vi "MGI Get Slope at Point.vi"(9 "Index":i32, 10 "Y[]":dbl[](array[numeric]), 11 "X[]":dbl[](array[numeric])) -> (3 "Slope Unit Vector[]":dbl[](array[numeric]))   [LabVIEW 2020]
doc: "Gets the unit length slope of the curve defined by the input arrays at the specified index.\n\nAuthored by Thomas E Henage\nsupport@mooregoodideas.com\nwww.mooregoodideas.com\n\nCopyright (c) 2010, Moore Good Ideas, Inc.\n\nAll rights reserved.\n\nRedistribution and use in source and binary forms, with or without modification, are permitted provided that the following conditions are met:\n\n * Redistributions of source code must retain the above copyright notice, this list of conditions and the following disclaimer.\n * Redistributions in binary form must reproduce the above copyright notice, this list of conditions and the following disclaimer in the documentation and/or other materials provided with the distribution.\n * Neither the name of Moore Good Ideas, Inc. nor the names of its contributors may be used to endorse or promote products derived from this software without specific prior written permission.\n\nTHIS SOFTWARE IS PROVIDED BY THE COPYRIGHT HOLDERS AND CONTRIBUTORS \"AS IS\" AND ANY EXPRESS OR IMPLIED WARRANTIES, INCLUDING, BUT NOT LIMITED TO, THE IMPLIED WARRANTIES OF MERCHANTABILITY AND FITNESS FOR A PARTICULAR PURPOSE ARE DISCLAIMED. IN NO EVENT SHALL THE COPYRIGHT OWNER OR CONTRIBUTORS BE LIABLE FOR ANY DIRECT, INDIRECT, INCIDENTAL, SPECIAL, EXEMPLARY, OR CONSEQUENTIAL DAMAGES (INCLUDING, BUT NOT LIMITED TO, PROCUREMENT OF SUBSTITUTE GOODS OR SERVICES; LOSS OF USE, DATA, OR PROFITS; OR BUSINESS INTERRUPTION) HOWEVER CAUSED AND ON ANY THEORY OF LIABILITY, WHETHER IN CONTRACT, STRICT LIABILITY, OR TORT (INCLUDING NEGLIGENCE OR OTHERWISE) ARISING IN ANY WAY OUT OF THE USE OF THIS SOFTWARE, EVEN IF ADVISED OF THE POSSIBILITY OF SUCH DAMAGE."
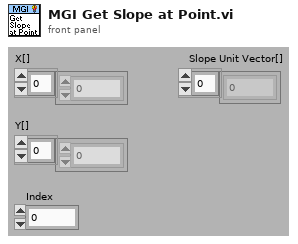
[diagram p1: front panel]
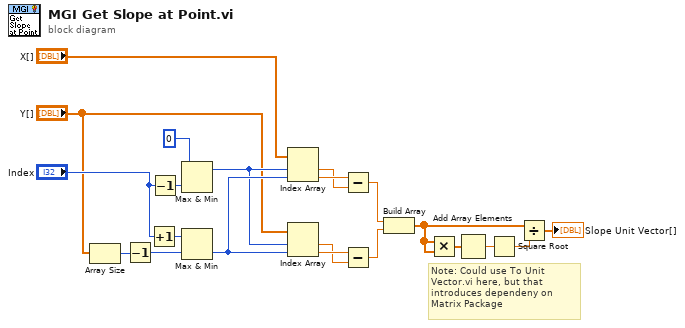
[diagram p0: block diagram]
diagram:
  # "Note: Could use To Unit Vector.vi here, but that introduces dependeny on Matrix Package"
  n1 = Array Size(array="Y[]") -> (size(s)=w6:i32)
  n2 = Decrement(x=w6) -> (x-1=w5:i32)
  n3 = Increment(x="Index") -> (x+1=w19:i32)
  n4 = Decrement(x="Index") -> (x-1=w16:i32)
  n5 = Max & Min(x=0, y=w16) -> (max(x,y)=w18:i32)  [unwired: 1 out]
  n6 = Max & Min(x=w19, y=w5) -> (min(x,y)=w20:i32)  [unwired: 1 out]
  n7 = Index Array(array="X[]", index #1=w18, index #2=w20) -> (element #1=w9:dbl, element #2=w15:dbl)
  n8 = Index Array(array="Y[]", index #1=w18, index #2=w20) -> (element #1=w10:dbl, element #2=w14:dbl)
  n9 = Subtract(x=w15, y=w9) -> (x-y=w11:dbl)
  n10 = Subtract(x=w14, y=w10) -> (x-y=w12:dbl)
  n11 = Build Array(w11, w12) -> (w4:dbl[])
  n12 = Multiply(x=w4, y=w4) -> (x*y=w3:dbl[])
  n13 = Add Array Elements(numeric array=w3) -> (sum=w2:dbl)
  n14 = Square Root(x=w2) -> (sqrt(x)=w1:dbl)
  n15 = Divide(x=w4, y=w1) -> (x/y=→"Slope Unit Vector[]":dbl[])
